vi "OAT Find RPM boundaries.vi"(5 "sampling frequency [Hz]":dbl=11025.0, 6 "speed profile":T1 {"speed [RPM]" format="%.2f"; "time [s]" format="%.2f"}, 7 "RPM range":T2 {"Increment" format="%.2f"; "Maximum" format="%.2f"; "Minimum" format="%.2f"}) -> (1 "RPM indices":i32[](array[numeric]), 3 "RPM boundaries":i32[](array[numeric]))   [LabVIEW 2017, in "SoundVib_Gabor.lvlib"]
uses:
  <vilib>/addons/Sound and Vibration/Order Analysis/Gabor Order Tracking/SoundVib_Gabor.lvlib
  <vilib>/addons/Sound and Vibration/Order Analysis/Tach Process/SubVIs/speed profile.ctl
  <vilib>/addons/Sound and Vibration/Order Analysis/Tach Process/SoundVib_TachProcess.lvlib
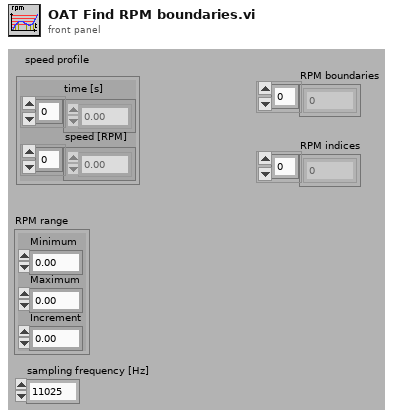
[diagram p1: front panel]
types:
  T1 = typedef "SoundVib_TachProcess.lvlib/speed profile.ctl" = cluster{"time [s]":dbl[], "speed [RPM]":dbl[]}
  T2 = cluster{"Minimum":dbl, "Maximum":dbl, "Increment":dbl}
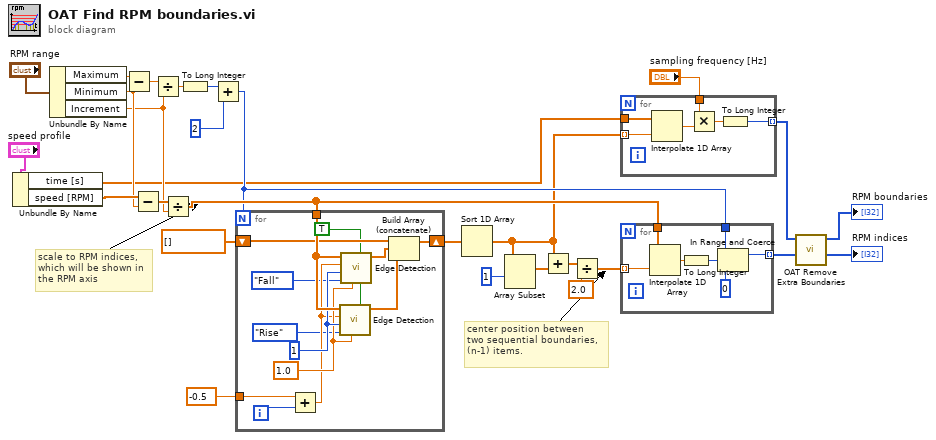
[diagram p0: block diagram]
diagram:
  # "scale to RPM indices, which will be shown in the RPM axis"
  # "center position between \ntwo sequential boundaries,\n(n-1) items."
  n1 = Unbundle By Name("speed profile") -> ("time [s]"=w6:dbl[], "speed [RPM]"=w26:dbl[])
  n2 = Unbundle By Name("RPM range") -> ("Maximum"=w24:dbl, "Minimum"=w23:dbl, "Increment"=w21:dbl)
  n3 = Subtract(x=w24, y=w23) -> (x-y=w22:dbl)
  n4 = Subtract(x=w26, y=w23) -> (x-y=w25:dbl[])
  n5 = Divide(x=w22, y=w21) -> (x/y=w15:dbl)
  n6 = Divide(x=w25, y=w21) -> (x/y=w20:dbl[])
  n7 = To Long Integer(number=w15) -> (32bit integer=w14:i32)
  n8 = Add(x=w14, y=2) -> (x+y=w19:i32)
  n9 = for {
    N: w19 -> [_]
    tunnel: w20 -> [w41]
    shift-right: [w38] -> w11
    shift-left: dbl[] [] -> [w39]
    tunnel: -0.5 -> [w34]
    i -> [w32]
    w29 = TRUE ("reset? (False)")
    w35 = 1.0 ("sampling frequency [Hz]")
    w40 = 1 ("pulse width (2)")
    n10 = Add(x=w34, y=w32) -> (x+y=w33:dbl)
    n11 = call <vilib>:"Edge Detection.vi"("reset? (True)"=w29, "sampling frequency [Hz]"=w35, "slope (Rise)"=enum16{"Rise", "Fall"}."Rise" ("slope (rise)"), "pulse width (2)"=w40, "threshold (0.0)"=w33, "x[n]"=w41) -> ("pulse positions [s]"=w36:dbl[])  [unwired: 4 in, 1 out]
    n12 = call <vilib>:"Edge Detection.vi"("reset? (True)"=w29, "sampling frequency [Hz]"=w35, "slope (Rise)"=enum16{"Rise", "Fall"}."Fall" ("slope (rise)"), "pulse width (2)"=w40, "threshold (0.0)"=w33, "x[n]"=w41) -> ("pulse positions [s]"=w37:dbl[])  [unwired: 4 in, 1 out]
    n13 = Build Array (concatenate)(w39, w37, w36) -> (w38:dbl[])
  }
  n14 = Sort 1D Array(array=w11) -> (sorted array=w7:dbl[])
  n15 = Array Subset(array=w7, index=1 ("Numeric")) -> (w10:dbl[])  [unwired: 1 in]
  n16 = Add(x=w7, y=w10) -> (x+y=w12:dbl[])
  n17 = Divide(x=w12, y=2.0 ("Numeric")) -> (x/y=w8:dbl[])
  n18 = for {
    tunnel: w7 -> [w47] mode=indexing
    tunnel: w6 -> [w46]
    tunnel: "sampling frequency [Hz]" -> [w43]
    tunnel: [w42] -> w4 mode=indexing
    n19 = Interpolate 1D Array(1:w47, 2:w46) -> (0:w45:dbl)
    n20 = Multiply(x=w43, y=w45) -> (x*y=w44:dbl)
    n21 = To Long Integer(number=w44) -> (32bit integer=w42:i32)
  }
  n22 = for {
    tunnel: w8 -> [w53] mode=indexing
    tunnel: w20 -> [w54]
    tunnel: w19 -> [w50]
    tunnel: [w49] -> w3 mode=indexing
    n23 = Interpolate 1D Array(1:w53, 2:w54) -> (0:w52:dbl)
    n24 = To Long Integer(number=w52) -> (32bit integer=w51:i32)
    n25 = In Range and Coerce(upper limit=w50, x=w51, lower limit=0) -> (coerced(x)=w49:i32)  [unwired: 1 out]
  }
  n26 = call <vilib>:"OAT Remove Extra Boundaries.vi"("RPM indices in"=w3, "time of RPM boundaries in"=w4) -> ("RPM indices out"=→"RPM indices":i32[], "time of RPM boundaries out"=→"RPM boundaries":i32[])  [unwired: 4 in]
